vi "Get_Client_ID.vi"(8 "error in (no error)":errorcluster, 11 "OneNote in":refnum<class "OneNote.lvclass">) -> (0 "error out":errorcluster, 3 "OneNote out":refnum<class "OneNote.lvclass">)   [LabVIEW 2016, in "OneNote.lvclass"]
uses:
  OneNote.lvclass
  OneNote.lvclass/OneNote.ctl
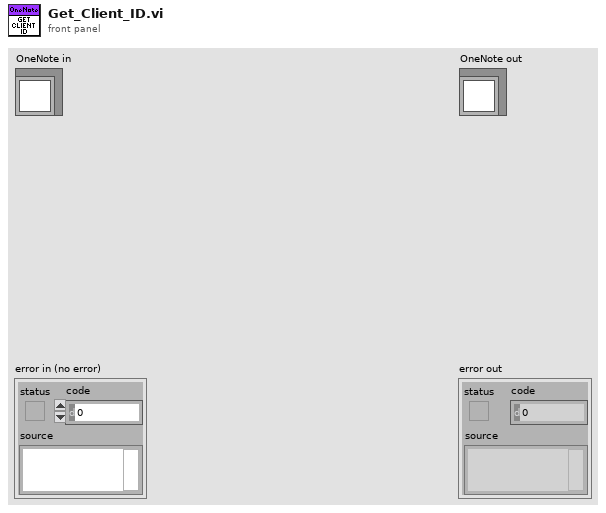
[diagram p1: front panel]
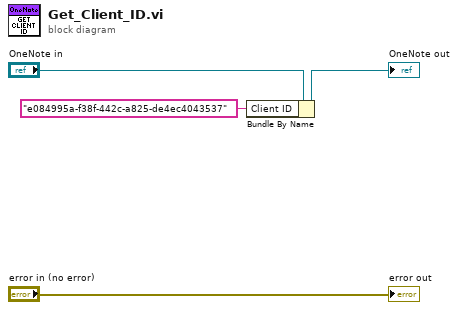
[diagram p0: block diagram]
diagram:
  n1 = Bundle By Name(cluster="OneNote in", "Client ID"="e084995a-f38f-442c-a825-de4ec4043537") -> (→"OneNote out":refnum<class "OneNote.lvclass">)
  "error out" <- "error in (no error)"
